vi "GetDeviceName.vi"(8 "error in (no error)":errorcluster, 11 "tdms file":refnum<k34>) -> (0 "error out":errorcluster, 2 "Device Name":string, 3 "tdms file out":refnum<k34>)   [LabVIEW 2015, in "Exposure Process.lvlib"]
uses:
  Exposure Process.lvlib
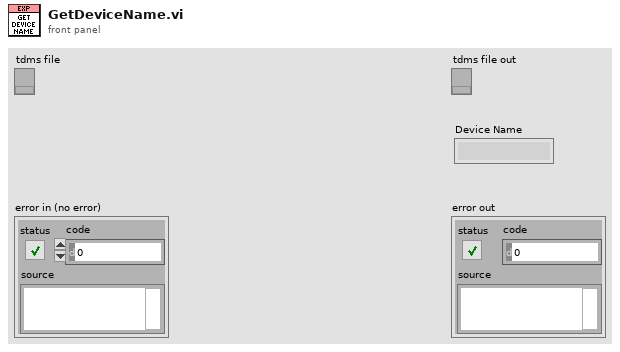
[diagram p1: front panel]
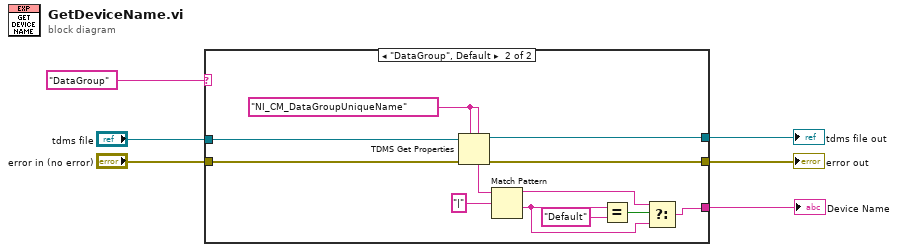
[diagram p0: block diagram]
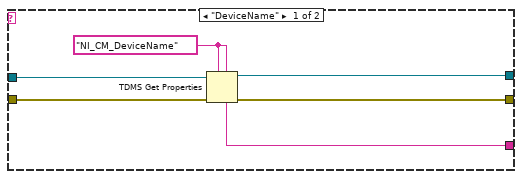
[diagram p2: hidden frame]
diagram:
  n1 = case shown="\"DataGroup\", Default" "DataGroup" {
    tunnel: "tdms file" -> [w11 w23]
    tunnel: "error in (no error)" -> [w10 w22]
    tunnel: [w9 w21] -> w4
    tunnel: [w8 w20] -> w3
    tunnel: [w7 w13] -> w1
    frame "DeviceName" {
      w12 = "NI_CM_DeviceName" ("property name")
      n2 = TDMS Get Properties(5:w12, 7:w12, 8:w10, 11:w11) -> (0:w8:errorcluster, 3:w9:refnum<k34>, 4:w7:string)  [unwired: 2 in, 3 out]
    }
    frame "DataGroup", Default {
      w24 = "NI_CM_DataGroupUniqueName" ("property name")
      n3 = TDMS Get Properties(5:w24, 7:w24, 8:w22, 11:w23) -> (0:w20:errorcluster, 3:w21:refnum<k34>, 4:w18:string)  [unwired: 2 in, 3 out]
      n4 = Match Pattern(string=w18, regular expression="|") -> (before substring=w15:string, after substring=w14:string)  [unwired: 1 in, 2 out]
      n5 = Equal?(x=w14, y="Default") -> (x = y?=w16:bool)
      n6 = Select(t=w15, s=w16, f=w14) -> (s? t:f=w13:string)
    }
  }
  "tdms file out" <- w4
  "error out" <- w3
  "Device Name" <- w1
